vi "Add Field to Image.vi"(7 "Justification":enum16{"Left", "Center", "Right"}(ring), 9 "Terminal Info":T1, 10 "location":i16=1, 11 "picture":picture) -> (1 "y":i16, 3 "new picture":picture)   [LabVIEW 2015, in "LVJSON.lvlib" / "Shared.lvlib"]
uses:
  Shared.lvlib
  Get Object Parameters/Parameter.ctl
  Get Object Parameters/offsets.vi
  Get Object Parameters/Get Object Parameters.xnode
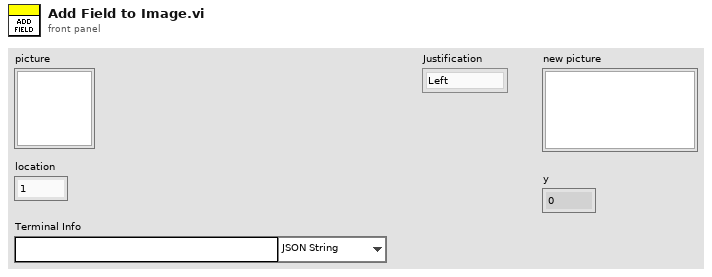
[diagram p1: front panel]
types:
  T1 = typedef "LVJSON.lvlib/Shared.lvlib/Parameter.ctl" = cluster{"Parameter Name":string, "JSON Type":enum16{"JSON String", "JSON Numeric", "JSON Boolean", "JSON", "JSON Object", "JSON Array", "String Value", "Numeric Value", "Boolean Value"}}
  T2 = enum16{"User-specified Font", "Application Font", "System Font", "Dialog Font"}
  T3 = cluster{"Font Name:":string, "Size":i16, "Strikeout?":bool, "Italic?":bool, "Underline?":bool, "Outline?":bool, "Shadow?":bool, "Bold?":bool}
  T4 = cluster{"left":i16, "top":i16, "right":i16, "bottom":i16}
  T5 = cluster{"horizontal":enum16{"left", "center", "right"}, "vertical":enum16{"top", "center", "bottom"}}
  T6 = enum16{"JSON String", "JSON Numeric", "JSON Boolean", "JSON", "JSON Object", "JSON Array", "String Value", "Numeric Value", "Boolean Value"}
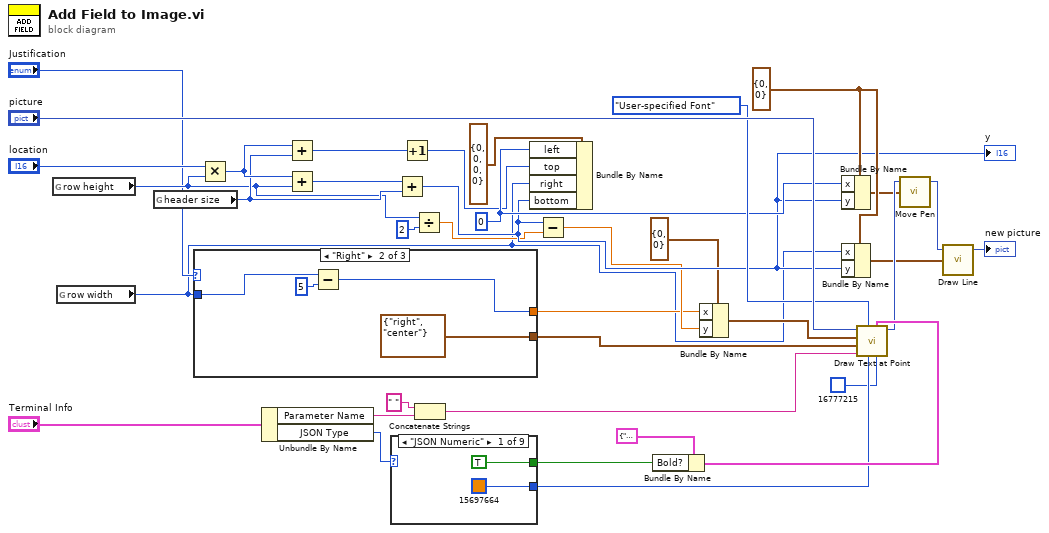
[diagram p0: block diagram]
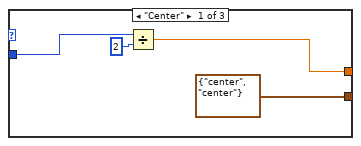
[diagram p2: hidden frame]
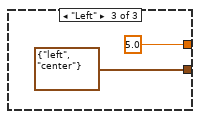
[diagram p3: hidden frame]
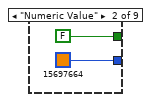
[diagram p4: hidden frame]
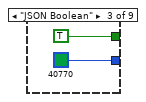
[diagram p5: hidden frame]
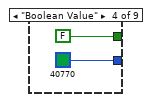
[diagram p6: hidden frame]
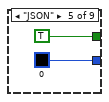
[diagram p7: hidden frame]
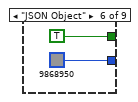
[diagram p8: hidden frame]
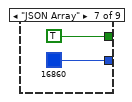
[diagram p9: hidden frame]
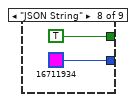
[diagram p10: hidden frame]
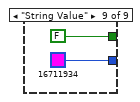
[diagram p11: hidden frame]
diagram:
  w16 = cluster{"x":i16, "y":i16} {"x"=0, "y"=0} ("end point")
  w17 = i16 0 ("left")
  n1 = global read "offsets.vi" "row height"() -> (w10:i16)
  n2 = global read "offsets.vi" "row width"() -> (w1:i16)
  n3 = global read "offsets.vi" "header size"() -> (w32:i16)
  n4 = case shown="\"Right\"" "Justification" {
    tunnel: [T5 {"horizontal"=enum."center", "vertical"=enum."center"} ("alignment(left, top)") T5 {"horizontal"=enum."right", "vertical"=enum."center"} ("alignment(left, top)") T5 {"horizontal"=enum."left", "vertical"=enum."center"} ("alignment(left, top)")] -> w3
    tunnel: [w39 w44 5.0 ("row width")] -> w2
    tunnel: w1 -> [w38 w43 _]
    frame "Center" {
      n5 = Divide(x=w38, y=i16 2) -> (x/y=w39:dbl)
    }
    frame "Right" {
      n6 = Subtract(x=w43, y=i16 5) -> (x-y=w44:i16)
    }
    frame "Left" {
    }
  }
  n7 = Multiply(x="location", y=w10) -> (x*y=w33:i16)
  n8 = Unbundle By Name("Terminal Info") -> ("Parameter Name"=w29:string, "JSON Type"=w23:T6)
  n9 = Add(x=w33, y=w32) -> (x+y=w13:i16)
  n10 = Add(x=w33, y=w10) -> (x+y=w34:i16)
  n11 = case shown="\"JSON Numeric\"" w23 {
    tunnel: [u32 15697664 ("text color(black)") u32 15697664 ("text color(black)") u32 40770 ("text color(black)") u32 40770 ("text color(black)") u32 0 ("text color(black)") u32 9868950 ("text color(black)") u32 16860 ("text color(black)") u32 16711934 ("text color(black)") u32 16711934 ("text color(black)")] -> w21
    tunnel: [TRUE FALSE TRUE FALSE TRUE TRUE TRUE TRUE FALSE] -> w22
    frame "JSON Numeric" {
    }
    frame "Numeric Value" {
    }
    frame "JSON Boolean" {
    }
    frame "Boolean Value" {
    }
    frame "JSON" {
    }
    frame "JSON Object" {
    }
    frame "JSON Array" {
    }
    frame "JSON String" {
    }
    frame "String Value" {
    }
  }
  n12 = Add(x=w34, y=w32) -> (x+y=w9:i16)
  "y" <- w9
  n13 = Increment(x=w13) -> (x+1=w12:i16)
  n14 = Divide(x=w10, y=i16 2) -> (x/y=w8:dbl)
  n15 = Concatenate Strings(" " ("string"), w29) -> (w28:string)
  n16 = Bundle By Name(cluster=T4 {"left"=0, "top"=0, "right"=0, "bottom"=0} ("rect"), "left"=w17, "top"=w12, "right"=w1, "bottom"=w9) -> ()  [unwired: 1 out]
  n17 = Subtract(x=w9, y=w8) -> (x-y=w7:dbl)
  n18 = Bundle By Name(cluster=T3 {"Font Name:"="Application", "Size"=15, "Strikeout?"=FALSE, "Italic?"=FALSE, "Underline?"=FALSE, "Outline?"=FALSE, "Shadow?"=FALSE, "Bold?"=FALSE} ("[user-specified font]"), "Bold?"=w22) -> (w25:T3)
  n19 = Bundle By Name(cluster=cluster{"x":i16, "y":i16} {"x"=0, "y"=0} ("input cluster"), "x"=w2, "y"=w7) -> (w5:cluster{"x":i16, "y":i16})
  n20 = Bundle By Name(cluster=w16, "x"=w17, "y"=w9) -> (w15:cluster{"x":i16, "y":i16})
  n21 = Bundle By Name(cluster=w16, "x"=w1, "y"=w9) -> (w14:cluster{"x":i16, "y":i16})
  n22 = call <vilib>:"Draw Text at Point.vi"("BG color(transparent)"=u32 16777215, "[user-specified font]"=w25, "text color(black)"=w21, "desired font(Application)"=T2."User-specified Font", "text"=w28, "alignment(left, top)"=w3, "origin"=w5, "picture"="picture") -> ("new picture"=w19:picture)  [unwired: 2 in, 1 out]
  n23 = call <vilib>:"Move Pen.vi"("new position"=w15, "picture"=w19) -> ("new picture"=w18:picture)  [unwired: 3 in]
  n24 = call <vilib>:"Draw Line.vi"("picture"=w18, "end point"=w14) -> ("new picture"=→"new picture":picture)  [unwired: 7 in]
